vi "Get Dispensed volume.vi"(7 "[x]":T1, 8 "error in (no error)":errorcluster, 11 "Serial Port in":refnum<visa-resource-name>) -> (0 "error out":errorcluster, 2 "Volume":dbl, 3 "Serial Port out":refnum<visa-resource-name>)   [LabVIEW 2020, in "Chemyx_Syringe_Pump_driver.lvlib"]
doc: "Returns the volume currently dispensed by the pump"
uses:
  Chemyx_Syringe_Pump_driver.lvlib
  _private/Control/Control Mode.ctl
panel:
  # "Returns the volume currently dispensed by the pump"
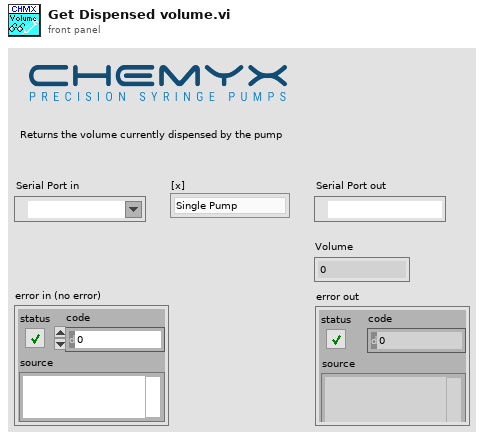
[diagram p1: front panel]
types:
  T1 = typedef "Chemyx_Syringe_Pump_driver.lvlib/Control Mode.ctl" = enum16{"Single Pump", "Pump Channel 1", "Pump Channel 2", "Cycle Mode"}
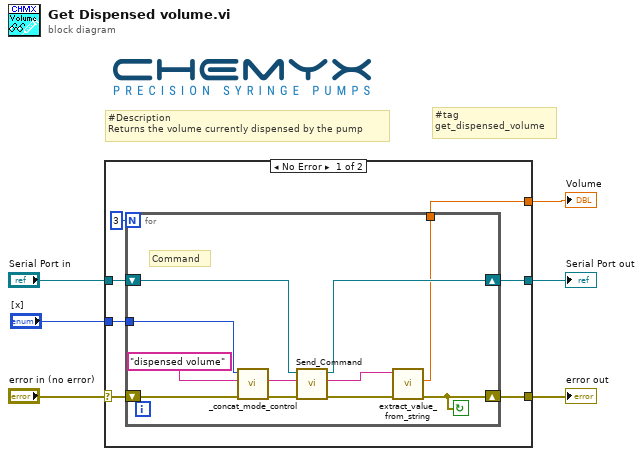
[diagram p0: block diagram]
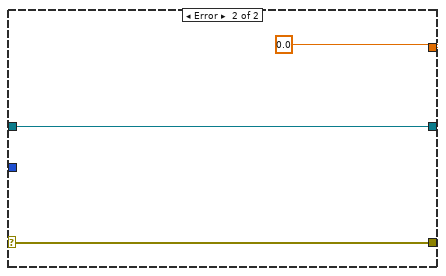
[diagram p2: hidden frame]
diagram:
  # "#tag\nget_dispensed_volume"
  # "#Description\nReturns the volume currently dispensed by the pump"
  n1 = case shown="No Error" "error in (no error)" {
    selector: "error in (no error)" -> [w12 w26]
    tunnel: "Serial Port in" -> [w13 w25]
    tunnel: [w10 w26] -> w4
    tunnel: [w11 w25] -> w3
    tunnel: [w9 0.0] -> w2
    tunnel: "[x]" -> [w8 _]
    frame No Error {
      n2 = for {
        N: 3 -> [_]
        tunnel: [w18] -> w9
        tunnel: w8 -> [w15]
        shift-right: [w21] -> w11
        shift-left: w13 -> [w23]
        shift-right: [w14] -> w10
        shift-left: w12 -> [w22]
        stop <- w14 continue-if-true
        # "Command"
        n3 = call "_concat_mode_control.vi"("write buffer"="dispensed volume", "[x]"=w15) -> ("write buffer out"=w16:string)  [unwired: 9 in]
        n4 = call "Send_Command.vi"("error in (no error)"=w22, "write buffer"=w16, "Serial Port in"=w23) -> ("error out"=w20:errorcluster, "Read buffer"=w19:string, "VISA Refnum out"=w21:refnum<visa-resource-name>)  [unwired: 6 in]
        n5 = call "extract_value_from_string.vi"("error in (no error)"=w20, "Input string"=w19) -> ("error out"=w14:errorcluster, "Value"=w18:dbl)  [unwired: 7 in, 1 out]
      }
    }
    frame Error {
    }
  }
  "error out" <- w4
  "Serial Port out" <- w3
  "Volume" <- w2
